vi "send udp and wait for slow response.vi"(8 "error in":errorcluster, 10 "command in":string="setwangle>>-0.644700000000", 11 "Device":string) -> (0 "error out":errorcluster, 2 "value":string, 3 "slow response":string)   [LabVIEW 2020]
uses:
  Shared/MySQL/Preset Query Enum.ctl
panel:
  in  "slow timeout ms (3000)":i32=3000
  out "Port Number":u16
  out "IP Address":string
  in  "Block Slow Port":bool
  out "ID fast":refnum<k16>
  in  "timeout ms (100)":i32=100
  # "setxyzuvw>>1,1,1,1,1,1"
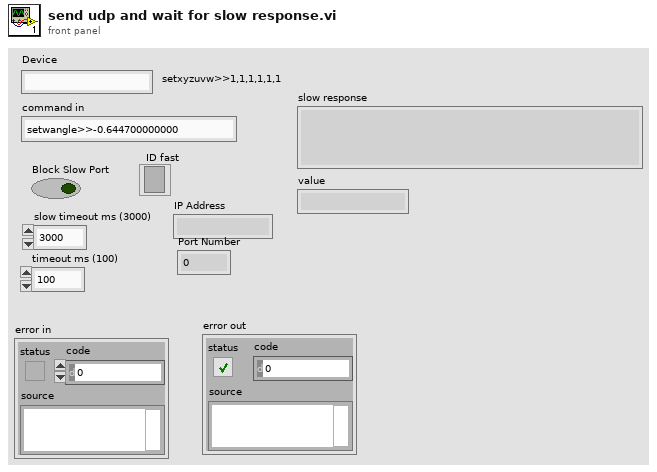
[diagram p1: front panel]
types:
  T1 = typedef "Preset Query Enum.ctl" = enum16{"Get Locations", "Get all IPs and MACs", "Get classes", "Get expt variables to set at scanstart for particular device", "Get expt devices and variables with start values", "Get expt devices and variables (with data to get)", "Get expt devices with data to get", "Get Expt devices and GUIs", "Get all devices basic properties", "Get Virtual Devices Core Info", "Get Expt names", "Get experiment basic properties", "Get experiment alarm variables", "Get MC Ports", "Get device network comm port", "Get devicetype lvclass path", "Get basic device properties", "Get Init Order", "Get all setable variables of a device", "Get device variable aliases", "Get force values of all settable variables", "Get all variables of a devicetype", "Get all variables of a device", "Get plotter details", "Get Saved Scans", "Get Scan Info", "GetGeneralGUIs", "Get expt for plotter", "Get plotter IDs from expt", "Get all devices", "Get all Virtual Devices", "Get all aliases", "Get variable and device info for Virtual Device", "GetItemLocatorIP", "Get IPs for GUIs", "Get DeviceType from Device", "GetLocalPortRange", "GetDevicePresetVariables", "Get Device Configuration", "GetAllPresetNames", "GetAllConfigurationNames", "GetPresetDeviceNames"}
  T2 = cluster{"data[0]":string, "data[1]":string, "data[2]":string, "data[3]":string, "data[4]":string, "data[5]":string, "data[6]":string, "data[7]":string, "data[8]":string}
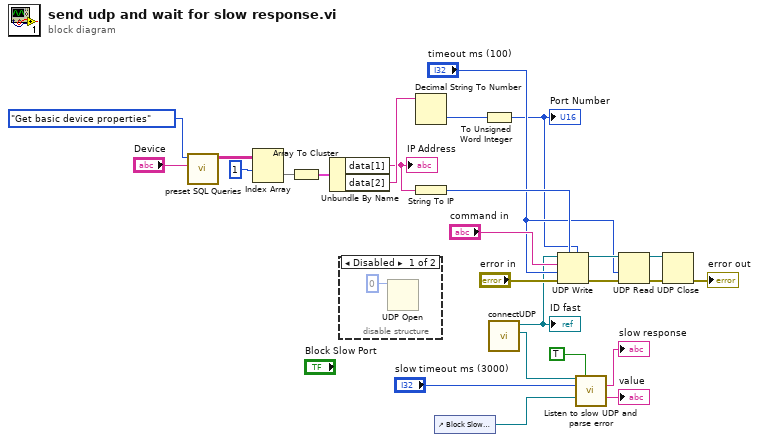
[diagram p0: block diagram]
diagram:
  n1 = call "preset SQL Queries.vi"("Device/Devicetype name\n/Plotter.id/ScanName#"="Device", "Preset Query"=Preset_Query_Enum."Get basic device properties") -> ("data"=w10:string[][])  [unwired: 7 in, 2 out]
  n2 = Index Array(array=w10, index (row)=1) -> (element=w8:string[])  [unwired: 1 in]
  n3 = Array To Cluster(array=w8) -> (cluster=w7:T2)
  n4 = Unbundle By Name(w7) -> ("data[1]"=w3:string, "data[2]"=w6:string)
  "IP Address" <- w3
  n5 = disable-structure shown="Disabled" {
    frame Disabled {
      n6 = UDP Open(11:u16 0 ("port")) -> ()  [unwired: 4 in, 3 out]
    }
    frame Enabled {
    }
  }
  n7 = Decimal String To Number(string=w6) -> (number=w5:i32)  [unwired: 2 in, 1 out]
  n8 = String To IP(1:w3) -> (0:w23:u32)
  n9 = control-ref of="Block Slow Port"() -> (w2:refnum<vi>)
  n10 = To Unsigned Word Integer(number=w5) -> (unsigned 16bit integer=w4:u16)
  "Port Number" <- w4
  n11 = call "connectUDP.vi"() -> ("fast ID (h)"=w1:refnum<k16>, "slow ID (h)"=w17:refnum<k16>)  [unwired: 1 in, 2 out]
  "ID fast" <- w1
  n12 = UDP Write(address=w23, port or service name=w4, connection ID=w1, data in="command in", 8:"error in", 9:"timeout ms (100)") -> (error out=w22:errorcluster, 3:w24:refnum<k16>)
  n13 = call "Listen to slow UDP and parse error.vi"("ID slow"=w17, "command accepted"=TRUE, "timeout ms (25000)"="slow timeout ms (3000)", "block slow port 2"=w2) -> ("data out"=→"slow response":string, "value"=→"value":string)  [unwired: 4 in, 6 out]
  n14 = UDP Read(connection ID=w24, timeout ms (25000)="timeout ms (100)", 8:w22) -> (error out=w20:errorcluster, 3:w19:refnum<k16>)  [unwired: 1 in, 3 out]
  n15 = UDP Close(connection ID=w19, 8:w20) -> (error out=→"error out":errorcluster)  [unwired: 1 out]
